vi "Report Server Manager Error.vi"(8 "error in (no error)":errorcluster, 10 "Server Manager Error":errorcluster, 11 "WS Test Server in":refnum<class "WS Test Server.lvclass">) -> (0 "error out":errorcluster, 3 "WS Test Server out":refnum<class "WS Test Server.lvclass">)   [LabVIEW 2021, in "Echo Broadcast with External Client.lvlib" / "WS Test Server.lvclass"]
uses:
  WS Test Server.lvclass
  WS Test Server.lvclass/WS Test Server.ctl
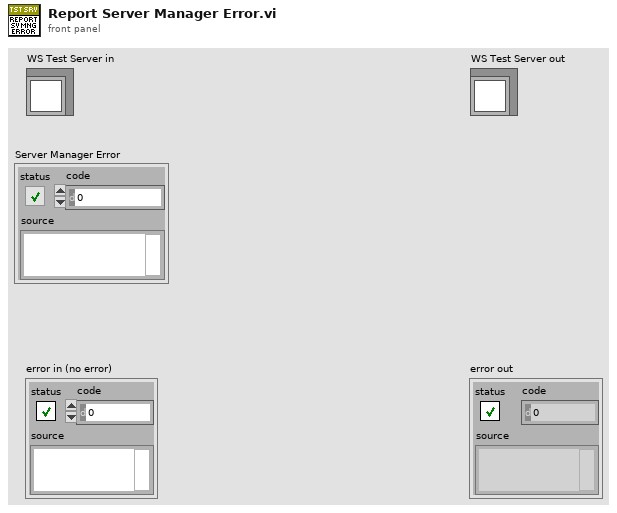
[diagram p1: front panel]
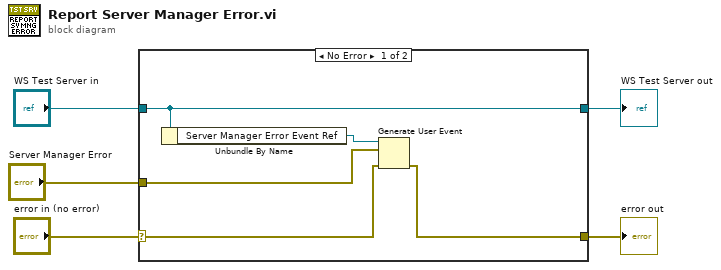
[diagram p0: block diagram]
diagram:
  n1 = case shown="No Error" "error in (no error)" {
    selector: "error in (no error)" -> [w7 w12]
    tunnel: [w6 w12] -> w4
    tunnel: [w10 w11] -> w2
    tunnel: "WS Test Server in" -> [w10 w11]
    tunnel: "Server Manager Error" -> [w8 _]
    frame No Error {
      n2 = Unbundle By Name(w10) -> ("Server Manager Error Event Ref"=w9:refnum<user-event>)
      n3 = Generate User Event(user event=w9, event data cluster=w8, error in=w7) -> (error out=w6:errorcluster)  [unwired: 1 in, 1 out]
    }
    frame Error {
    }
  }
  "error out" <- w4
  "WS Test Server out" <- w2
